vi "Write Trigger_TargetsRef.vi"(8 "error in (no error)":errorcluster, 10 "Trigger_TargetsRef":refnum<vi>, 11 "Electronic Load in":refnum<class "Electronic Load.lvclass">) -> (0 "error out":errorcluster, 3 "Electronic Load out":refnum<class "Electronic Load.lvclass">)   [LabVIEW 2019, in "Electronic Load.lvlib" / "Electronic Load.lvclass"]
uses:
  Library/Electronic Load.lvclass
  Library/Electronic Load.lvclass/Electronic Load.ctl
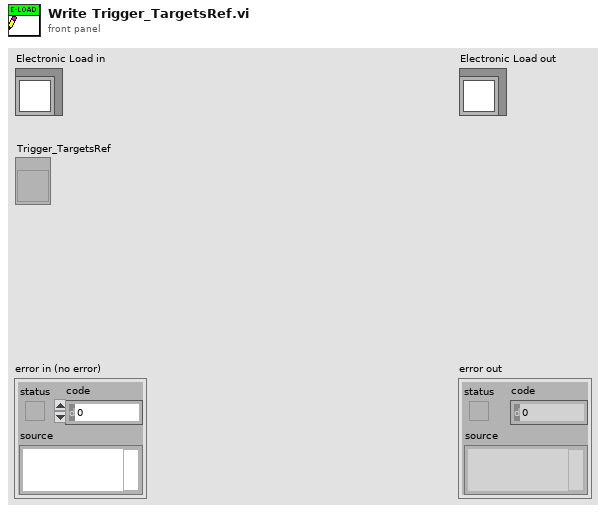
[diagram p1: front panel]
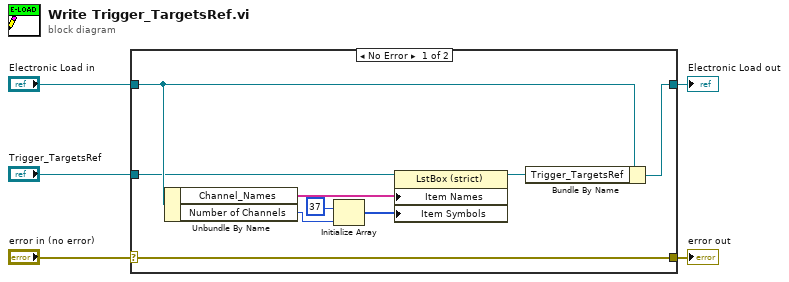
[diagram p0: block diagram]
diagram:
  n1 = case shown="No Error" "error in (no error)" {
    selector: "error in (no error)" -> [w14 w15]
    tunnel: [w14 w15] -> w4
    tunnel: [w13 w16] -> w2
    tunnel: "Electronic Load in" -> [w12 w16]
    tunnel: "Trigger_TargetsRef" -> [w11 _]
    frame No Error {
      n2 = Unbundle By Name(w12) -> ("Channel_Names"=w9:string[], "Number of Channels"=w8:i32)
      n3 = Initialize Array(37, w8) -> (w7:i32[])
      n4 = property class="LstBox (strict)"(reference=w11, "Item Names"=w9, "Item Symbols"=w7) -> (reference out=w10:refnum<vi>)  [unwired: 1 in, 1 out]
      n5 = Bundle By Name(cluster=w12, "Trigger_TargetsRef"=w10) -> (w13:refnum<class "Electronic Load.lvclass">)
    }
    frame Error {
    }
  }
  "error out" <- w4
  "Electronic Load out" <- w2
